vi "Copy Gantry Data.vi"(8 "error in (no error)":errorcluster, 10 "Gantry Source":refnum<class "Gantry Class.lvclass">, 11 "Gantry Dest":refnum<class "Gantry Class.lvclass">) -> (0 "error out":errorcluster, 3 "Gantry Result":refnum<class "Gantry Class.lvclass">)   [LabVIEW 2011]
uses:
  Gantry Class/Gantry Class.lvclass
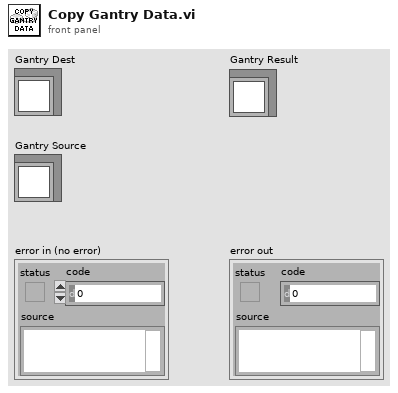
[diagram p1: front panel]
types:
  T1 = typedef "Gantry_Camera.ctl" = cluster{"Name":string, "IMAQ Session":T2, "Group":u32, "Open?":bool, "Interface Name":string}
  T2 = typedef "IMAQdx.ctl" = refnum<k21>
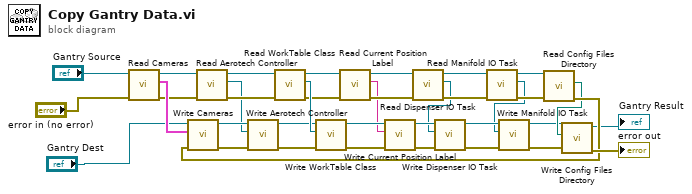
[diagram p0: block diagram]
diagram:
  n1 = call-dynamic "Read Cameras.vi"("error in (no error)"="error in (no error)", "Gantry Class in"="Gantry Source") -> ("error out"=w4:errorcluster, "Cameras"=w14:T1[], "Gantry Class out"=w3:refnum<class "Gantry Class.lvclass">)  [unwired: 7 in]
  n2 = call-dynamic "Read Aerotech Controller.vi"("error in (no error)"=w4, "Gantry Class in"=w3) -> ("error out"=w5:errorcluster, "Aerotech Controller"=w2:refnum<k24>, "Gantry Class out"=w6:refnum<class "Gantry Class.lvclass">)  [unwired: 7 in]
  n3 = call-dynamic "Read WorkTable Class.vi"("error in"=w5, "Gantry Class in"=w6) -> ("error out"=w7:errorcluster, "WorkTable Class.lvclass"=w18:refnum<class "WorkTable Class.lvclass">, "Gantry Class out"=w10:refnum<class "Gantry Class.lvclass">)  [unwired: 7 in]
  n4 = call-dynamic "Read Current Position Label.vi"("error in (no error)"=w7, "Gantry Class in"=w10) -> ("error out"=w8:errorcluster, "Current Position Label"=w1:string, "Gantry Class out"=w9:refnum<class "Gantry Class.lvclass">)  [unwired: 7 in]
  n5 = call-dynamic "Read Dispenser IO Task.vi"("error in (no error)"=w8, "Gantry Class in"=w9) -> ("error out"=w31:errorcluster, "Dispenser IO Task"=w23:refnum<k21>, "Gantry Class out"=w22:refnum<class "Gantry Class.lvclass">)  [unwired: 7 in]
  n6 = call-dynamic "Read Manifold IO Task.vi"("error in (no error)"=w31, "Gantry Class in"=w22) -> ("error out"=w32:errorcluster, "Manifold IO Task"=w24:refnum<k21>, "Gantry Class out"=w27:refnum<class "Gantry Class.lvclass">)  [unwired: 7 in]
  n7 = call-dynamic "Read Config Files Directory.vi"("error in (no error)"=w32, "Gantry Class in"=w27) -> ("error out"=w33:errorcluster, "Config Files Directory"=w29:path)  [unwired: 7 in, 1 out]
  n8 = call-dynamic "Write Cameras.vi"("error in (no error)"=w33, "Cameras"=w14, "Gantry Class in"="Gantry Dest") -> ("error out"=w15:errorcluster, "Gantry Class out"=w16:refnum<class "Gantry Class.lvclass">)  [unwired: 7 in]
  n9 = call-dynamic "Write Aerotech Controller.vi"("error in (no error)"=w15, "Aerotech Controller"=w2, "Gantry Class in"=w16) -> ("error out"=w19:errorcluster, "Gantry Class out"=w17:refnum<class "Gantry Class.lvclass">)  [unwired: 7 in]
  n10 = call-dynamic "Write WorkTable Class.vi"("error in (no error)"=w19, "WorkTable Class.lvclass"=w18, "Gantry Class in"=w17) -> ("error out"=w21:errorcluster, "Gantry Class out"=w20:refnum<class "Gantry Class.lvclass">)  [unwired: 7 in]
  n11 = call-dynamic "Write Current Position Label.vi"("error in (no error)"=w21, "Current Position Label"=w1, "Gantry Class in"=w20) -> ("error out"=w34:errorcluster, "Gantry Class out"=w25:refnum<class "Gantry Class.lvclass">)  [unwired: 7 in]
  n12 = call-dynamic "Write Dispenser IO Task.vi"("error in (no error)"=w34, "Dispenser IO Task"=w23, "Gantry Class in"=w25) -> ("error out"=w35:errorcluster, "Gantry Class out"=w26:refnum<class "Gantry Class.lvclass">)  [unwired: 7 in]
  n13 = call-dynamic "Write Manifold IO Task.vi"("error in (no error)"=w35, "Manifold IO Task"=w24, "Gantry Class in"=w26) -> ("error out"=w36:errorcluster, "Gantry Class out"=w28:refnum<class "Gantry Class.lvclass">)  [unwired: 7 in]
  n14 = call-dynamic "Write Config Files Directory.vi"("error in (no error)"=w36, "Config Files Directory"=w29, "Gantry Class in"=w28) -> ("error out"=→"error out":errorcluster, "Gantry Class out"=→"Gantry Result":refnum<class "Gantry Class.lvclass">)  [unwired: 7 in]
